vi "Read Test Suite Result.vi"(8 "error in (no error)":errorcluster, 11 "Test Assert Factory in":refnum<class "Test Assert Factory.lvclass">) -> (0 "error out":errorcluster, 2 "Test Suite Result":refnum<user-event>, 3 "Test Assert Factory out":refnum<class "Test Assert Factory.lvclass">)   [LabVIEW 2013, in "Caraya.lvlib" / "Test Assert Factory.lvclass"]
uses:
  Test Assert Factory.lvclass
  Test Result/Test Result.lvclass
  Test Assert Factory.lvclass/Test Assert Factory.ctl
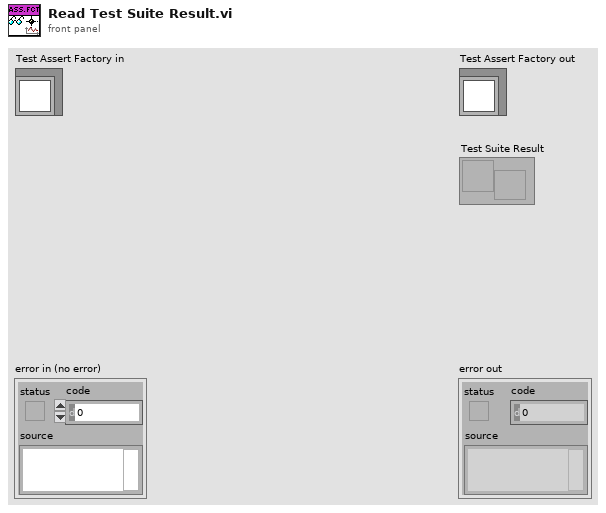
[diagram p1: front panel]
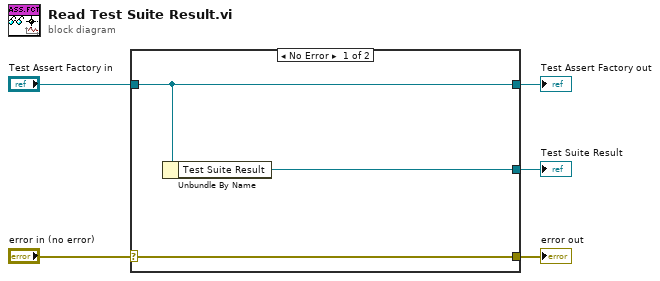
[diagram p0: block diagram]
diagram:
  n1 = case shown="No Error" "error in (no error)" {
    selector: "error in (no error)" -> [w8 w9]
    tunnel: [w8 w9] -> w4
    tunnel: [w7 w10] -> w2
    tunnel: "Test Assert Factory in" -> [w7 w10]
    tunnel: [w6 _] -> w1
    frame No Error {
      n2 = Unbundle By Name(w7) -> ("Test Suite Result"=w6:refnum<user-event>)
    }
    frame Error {
    }
  }
  "error out" <- w4
  "Test Assert Factory out" <- w2
  "Test Suite Result" <- w1
